vi "ACT LG Activity Log Core.vi"(0 "Object In":T1={"Log Size (Lines)"=450, "Log Path"=path "logfiles/Detailed Log", "Display Refs"=[]}, 1 "Display Ref":refnum<vi>, 5 "Source":string, 7 "Log Line":string, 11 "Error In (no error)":errorcluster, 13 "Log (T)":bool=TRUE) -> (8 "Timestamp":string, 15 "Error Out":errorcluster)   [LabVIEW 2012]
uses:
  Type Defs/ACT LG Parameters Cluster.ctl
  File IO/Type Defs/FILE New Line Enum.ctl
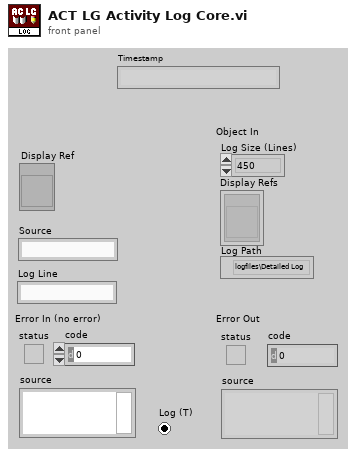
[diagram p1: front panel]
types:
  T1 = typedef "ACT LG Parameters Cluster.ctl" = cluster{"Log Size (Lines)":i32, "Log Path":path, "Display Refs":refnum<vi>[]}
  T2 = typedef "FILE New Line Enum.ctl" = enum16{"No New Line", "New Line"}
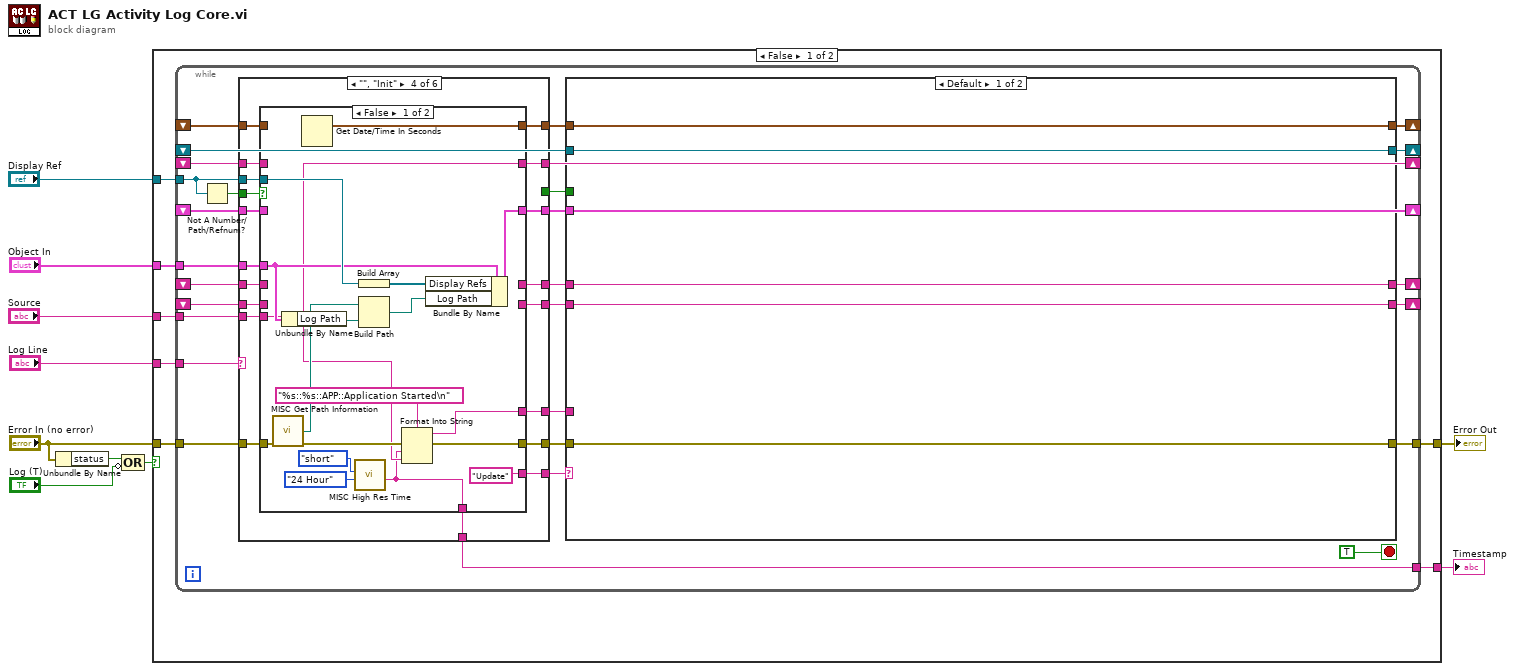
[diagram p0: block diagram]
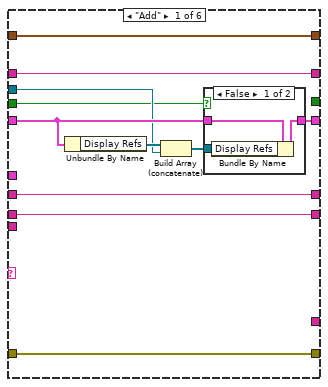
[diagram p2: hidden frame]
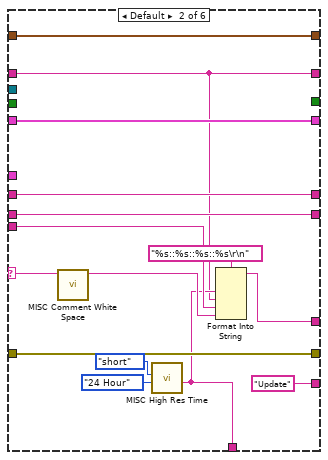
[diagram p4: hidden frame]
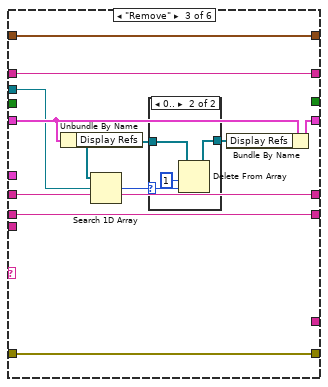
[diagram p5: hidden frame]
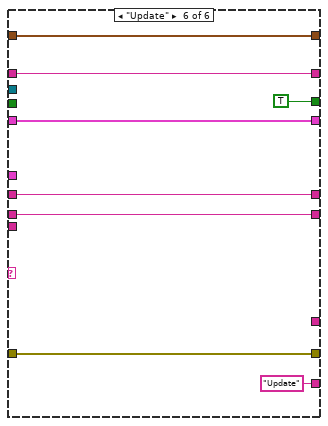
[diagram p9: hidden frame]
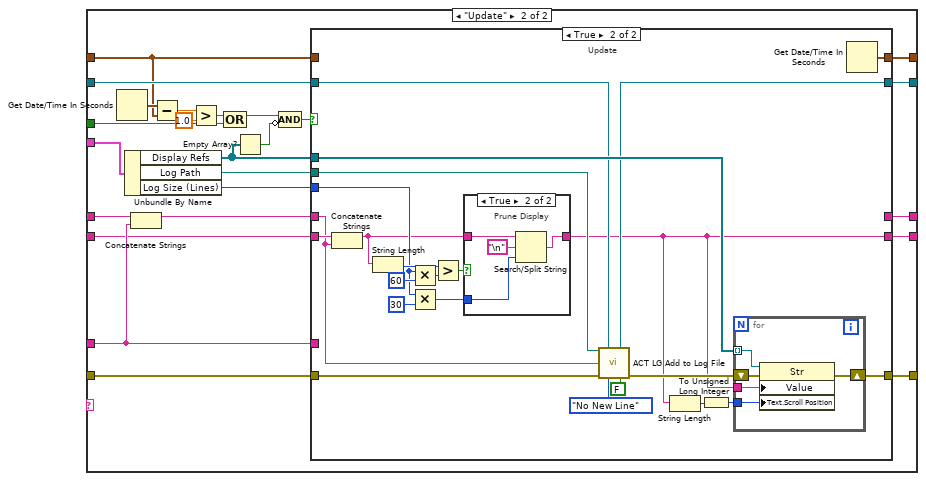
[diagram p10: hidden frame]
diagram:
  n1 = Unbundle By Name("Error In (no error)") -> ("status"=w4:bool)
  n2 = Compound Arithmetic op=OR(w4, invert "Log (T)") -> (w2:bool)
  n3 = case shown="False" w2 {
    tunnel: [w16 w216] -> w10
    tunnel: "Log Line" -> [w17 _]
    tunnel: "Object In" -> [w15 _]
    tunnel: "Source" -> [w14 _]
    tunnel: "Display Ref" -> [w13 _]
    tunnel: [w12 _] -> w5
    tunnel: "Error In (no error)" -> [w11 w216]
    frame False {
      n4 = while {
        tunnel: w11 -> [w44]
        tunnel: w17 -> [w36]
        tunnel: [w42] -> w16
        tunnel: w15 -> [w38]
        shift-right: [w41] -> _
        shift-left: _ -> [w43]
        shift-right: [w37] -> _
        shift-left: _ -> [w39]
        tunnel: w14 -> [w35]
        tunnel: w13 -> [w34]
        shift-right: [w29] -> _
        shift-left: _ -> [w30]
        shift-right: [w28] -> _
        shift-left: _ -> [w26]
        shift-right: [w23] -> _
        shift-left: _ -> [w25]
        tunnel: [w20] -> w12
        shift-right: [w19] -> _
        shift-left: _ -> [w18]
        stop <- TRUE stop-if-true
        n5 = Not A Number/Path/Refnum?(number/path/refnum=w34) -> (NaN/Path/Refnum?=w31:bool)
        n6 = case shown="\"\", \"Init\"" w36 {
          selector: w36 -> [_ w64 _ _ _ _]
          tunnel: [w55 w75 w85 w110 w140 w148] -> w40
          tunnel: [_ w69 _ w109 _ _] -> w33
          tunnel: w44 -> [w55 w75 w85 w108 w140 w148]
          tunnel: w34 -> [w51 _ w83 w107 _ _]
          tunnel: w39 -> [w54 w74 w84 w103 w139 w147]
          tunnel: [w56 w74 w86 w106 w139 w147] -> w37
          tunnel: w38 -> [_ _ _ w105 _ _]
          tunnel: w43 -> [w49 w70 w79 w102 w138 w146]
          tunnel: w35 -> [_ w68 _ w94 _ _]
          tunnel: [w49 w70 w79 w101 w138 w146] -> w45
          tunnel: w31 -> [w50 _ _ w104 _ _]
          tunnel: [w48 w67 w78 w100 w137 w145] -> w27
          tunnel: w26 -> [w48 w67 w78 w99 w137 w145]
          tunnel: [w47 w66 w77 w97 w136 w144] -> w24
          tunnel: w25 -> [w47 w66 w77 w98 w136 w144]
          tunnel: [_ _ _ _ _ TRUE] -> w22
          tunnel: [_ "Update" _ w96 _ "Update"] -> w21
          tunnel: [_ w62 _ w95 _ _] -> w20
          tunnel: [w46 w61 w76 w93 w135 w141] -> w19
          tunnel: w18 -> [w46 w61 w76 w92 w135 w141]
          frame "Add" {
            n7 = Unbundle By Name(w54) -> ("Display Refs"=w53:refnum<vi>[])
            n8 = Build Array (concatenate)(w53, w51) -> (w52:refnum<vi>[])
            n9 = case shown="False" w50 {
              tunnel: [w59 w60] -> w56
              tunnel: w54 -> [w58 w60]
              tunnel: w52 -> [w57 _]
              frame False {
                n10 = Bundle By Name(cluster=w58, "Display Refs"=w57) -> (w59:T1)
              }
              frame True {
              }
            }
          }
          frame Default {
            n11 = call "MISC Comment White Space.vi"("Input String"=w64) -> ("Output String"=w63:string)  [unwired: 10 out]
            n12 = call "MISC High Res Time.vi"("Time Standard (am/pm)"=enum16{"AM/PM", "24 Hour"}."24 Hour", "Date Format (Abb)"=enum16{"short", "long", "abbreviated"}."short" ("date format (abbreviated)")) -> ("Date/Time String"=w62:string)  [unwired: 1 in, 6 out]
            n13 = Format Into String(format string="%s::%s::%s::%s\r\n", w62, w61, w68, w63) -> (resulting string=w69:string)  [unwired: 2 in, 1 out]
          }
          frame "Remove" {
            n14 = Unbundle By Name(w84) -> ("Display Refs"=w80:refnum<vi>[])
            n15 = Search 1D Array(1D array=w80, element=w83) -> (index of element=w82:i32)  [unwired: 1 out]
            n16 = case shown="0.." w82 {
              selector: w82 -> [_ w91]
              tunnel: [w87 w89] -> w81
              tunnel: w80 -> [w87 w88]
              frame ..-1 {
              }
              frame 0.. {
                n17 = Delete From Array(array=w88, length=1, index=w91) -> (array with subset deleted=w89:refnum<vi>[])  [unwired: 1 out]
              }
            }
            n18 = Bundle By Name(cluster=w84, "Display Refs"=w81) -> (w86:T1)
          }
          frame "", "Init" {
            n19 = case shown="False" w104 {
              tunnel: [w125 w133] -> w110
              tunnel: [w124 _] -> w109
              tunnel: w108 -> [w119 w133]
              tunnel: w107 -> [w123 _]
              tunnel: [w122 w134] -> w106
              tunnel: w105 -> [w120 _]
              tunnel: w103 -> [_ w134]
              tunnel: [_ w132] -> w101
              tunnel: w102 -> [_ w132]
              tunnel: [w114 w131] -> w100
              tunnel: w99 -> [_ w131]
              tunnel: [_ w130] -> w97
              tunnel: w98 -> [_ w130]
              tunnel: ["Update" _] -> w96
              tunnel: [w111 _] -> w95
              tunnel: w94 -> [w112 _]
              tunnel: [w112 w129] -> w93
              tunnel: w92 -> [_ w129]
              frame False {
                n20 = call "MISC Get Path Information.vi"("Error In (no error)"=w119) -> ("Support Directory"=w117:path, "Error Out"=w118:errorcluster)  [unwired: 13 out]
                n21 = Unbundle By Name(w120) -> ("Log Path"=w116:path)
                n22 = Get Date/Time In Seconds() -> (seconds since 1Jan1904=w114:timestamp)
                n23 = call "MISC High Res Time.vi"("Time Standard (am/pm)"=enum16{"AM/PM", "24 Hour"}."24 Hour", "Date Format (Abb)"=enum16{"short", "long", "abbreviated"}."short" ("date format (abbreviated)")) -> ("Date/Time String"=w111:string)  [unwired: 1 in, 6 out]
                n24 = Build Array(w123) -> (w121:refnum<vi>[])
                n25 = Build Path(base path=w117, name or relative path=w116) -> (appended path=w115:path)
                n26 = Format Into String(format string="%s::%s::APP::Application Started\n", error in=w118, w111, w112) -> (resulting string=w124:string, error out=w125:errorcluster)  [unwired: 1 in]
                n27 = Bundle By Name(cluster=w120, "Display Refs"=w121, "Log Path"=w115) -> (w122:T1)
              }
              frame True {
              }
            }
          }
          frame "Close" {
          }
          frame "Update" {
          }
        }
        n28 = case shown="Default" w21 {
          tunnel: w45 -> [w153 w165]
          tunnel: [w152 w177] -> w42
          tunnel: [w153 w164] -> w41
          tunnel: w40 -> [w152 w171]
          tunnel: w33 -> [_ w172]
          tunnel: w37 -> [_ w175]
          tunnel: w30 -> [w151 w174]
          tunnel: [w151 w173] -> w29
          tunnel: [w149 w158] -> w28
          tunnel: w27 -> [w149 w159]
          tunnel: w24 -> [w150 w167]
          tunnel: [w150 w163] -> w23
          tunnel: w22 -> [_ w160]
          frame Default {
          }
          frame "Update" {
            n29 = Get Date/Time In Seconds() -> (seconds since 1Jan1904=w170:timestamp)
            n30 = Unbundle By Name(w175) -> ("Display Refs"=w154:refnum<vi>[], "Log Path"=w176:path, "Log Size (Lines)"=w166:i32)
            n31 = Concatenate Strings(w167, w172) -> (w162:string)
            n32 = Subtract(x=w170, y=w159) -> (x-y=w169:dbl)
            n33 = Greater?(x=w169, y=1.0) -> (0:w161:bool)
            n34 = Compound Arithmetic op=OR(w161, w160) -> (w157:bool)
            n35 = Empty Array?(array=w154) -> (empty?=w155:bool)
            n36 = Compound Arithmetic op=AND(w157, invert w155) -> (w156:bool)
            n37 = case shown="True" w156 {
              tunnel: [w178 w203] -> w177
              tunnel: w154 -> [_ w202]
              tunnel: w165 -> [w182 w186]
              tunnel: w176 -> [_ w200]
              tunnel: w174 -> [w179 w199]
              tunnel: [w179 w198] -> w173
              tunnel: w172 -> [_ _]
              tunnel: w171 -> [w178 w195]
              tunnel: w166 -> [_ w188]
              tunnel: [w182 w187] -> w164
              tunnel: w162 -> [w181 w185]
              tunnel: [w181 _] -> w163
              tunnel: [w180 w183] -> w158
              tunnel: w159 -> [w180 _]
              frame False {
              }
              frame True {
                # "Update"
                n38 = Concatenate Strings(w186, w185) -> (w184:string)
                n39 = String Length(string=w184) -> (length=w192:i32)
                n40 = Multiply(x=w188, y=60) -> (x*y=w190:i32)
                n41 = Multiply(x=w188, y=30) -> (x*y=w194:i32)
                n42 = Greater?(x=w192, y=w190) -> (0:w191:bool)
                n43 = case shown="True" w191 {
                  tunnel: [w206 w208] -> w187
                  tunnel: w184 -> [w206 w210]
                  tunnel: w194 -> [_ w207]
                  frame False {
                  }
                  frame True {
                    # "Prune Display"
                    n44 = Search/Split String(string=w210, search string/char (-)="\n", offset (0)=w207) -> (match + rest of string=w208:string)  [unwired: 2 out]
                  }
                }
                n45 = call "ACT LG Add to Log File.vi"("Directory Log Path"=w200, "File Refnum In"=w199, "Line To Append"=w185, "Error in (no error)"=w195, "Append Mode (new line)"=FILE_New_Line_Enum."No New Line" ("new line on append? (new line)"), "Timestamp (t:yes)"=FALSE ("Include Timestamp (t:yes)")) -> ("File Refnum Out"=w198:refnum<file>, "Error out"=w201:errorcluster)  [unwired: 2 in, 6 out]
                n46 = String Length(string=w187) -> (length=w204:i32)
                n47 = To Unsigned Long Integer(number=w204) -> (unsigned 32bit integer=w205:u32)
                n48 = for {
                  tunnel: w205 -> [w215]
                  tunnel: w202 -> [w213] mode=indexing
                  tunnel: w187 -> [w211]
                  shift-right: [w214] -> w203
                  shift-left: w201 -> [w212]
                  n49 = property class="Str"(reference=w213, error in=w212, "Value"=w211, "Text.Scroll Position"=w215) -> (error out=w214:errorcluster)  [unwired: 1 out]
                }
                n50 = Get Date/Time In Seconds() -> (seconds since 1Jan1904=w183:timestamp)
              }
            }
          }
        }
      }
    }
    frame True {
      (unwired) FALSE ("Acquired Out")
    }
  }
  "Error Out" <- w10
  "Timestamp" <- w5
